vi "ums_to_I16tick.vi"(5 "Positions":dbl[](array[numeric])=[0.0, 0.0], 6 "Max piezo distance":dbl, 7 "n":u32=27, 8 "-10 to +10V?":bool, 9 "Input Velocity":dbl[](array[numeric])=[10.0]) -> (0 "Error":bool, 3 "Scalled Velocity":i16[](array[numeric]))   [LabVIEW 2023]
uses:
  User_Vi/Settings.vi
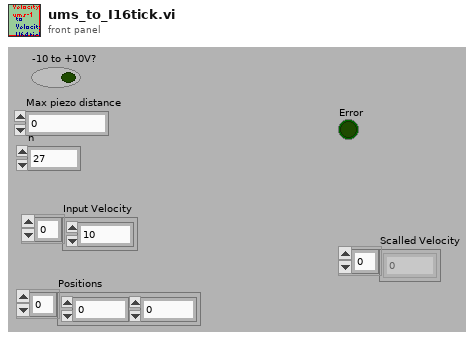
[diagram p1: front panel]
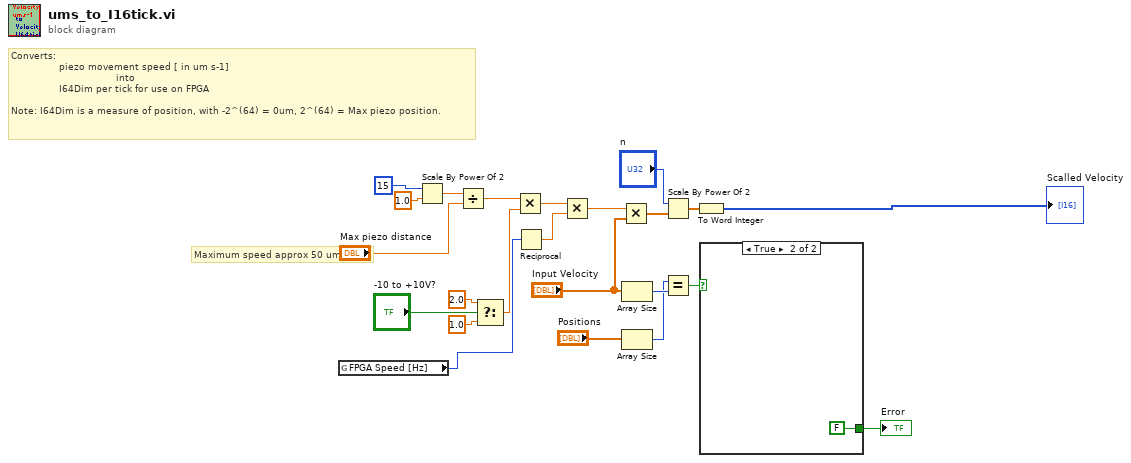
[diagram p0: block diagram]
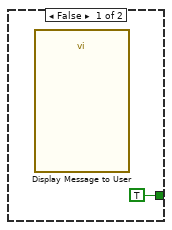
[diagram p2: hidden frame]
diagram:
  # "Maximum speed approx 50 um/s"
  # "Converts:\n                piezo movement speed [ in um s-1]\n                                   into\n                I64Dim per tick for use on FPGA\n\nNote: I64Dim is a measure of position, with -2^(64) = 0um, 2^(64) = Max piezo position."
  n1 = global read "Settings.vi" "FPGA Speed [Hz]"() -> (w1:i64)
  n2 = Scale By Power Of 2(n=i16 15, x=1.0) -> (x*2^n=w14:dbl)
  n3 = Divide(x=w14, y="Max piezo distance") -> (x/y=w4:dbl)
  n4 = Select(t=2.0 ("f"), s="-10 to +10V?", f=1.0) -> (s? t:f=w7:dbl)
  n5 = Multiply(x=w4, y=w7) -> (x*y=w3:dbl)
  n6 = Reciprocal(x=w1) -> (1/x=w17:dbl)
  n7 = Multiply(x=w3, y=w17) -> (x*y=w13:dbl)
  n8 = Multiply(x=w13, y="Input Velocity") -> (x*y=w9:dbl[])
  n9 = Array Size(array="Input Velocity") -> (size(s)=w22:i32)
  n10 = Array Size(array="Positions") -> (size(s)=w18:i32)
  n11 = Scale By Power Of 2(n="n", x=w9) -> (x*2^n=w11:dbl[])
  n12 = Equal?(x=w18, y=w22) -> (x = y?=w21:bool)
  n13 = To Word Integer(number=w11) -> (16bit integer=→"Scalled Velocity":i16[])
  n14 = case shown="True" w21 {
    tunnel: [TRUE FALSE] -> w20
    frame False {
      n15 = call "Display Message to User"() -> ()  [unwired: 10 in, 2 out]
    }
    frame True {
    }
  }
  "Error" <- w20
